vi "turn.vi"(8 "Angle":dbl=45.0 format="%#_13g", 10 "y":dbl=-1.0, 11 "RobotDriveDevRef":T1={"DevStatus"={"status"=FALSE, "code"=0, "source"=""}, "Motors[]"=[], "Square Inputs"=FALSE, "Max Output"=1.0}) -> (3 "RobotDriveDevRef dup.":T1={"DevStatus"={"status"=FALSE, "code"=0, "source"=""}, "Motors[]"=[], "Square Inputs"=FALSE, "Max Output"=1.0})   [LabVIEW 2016]
uses:
  <vilib>/Rock Robotics/WPI/RobotDrive/WPI_RobotDriveDevRef.ctl
  <vilib>/Rock Robotics/WPI/MotorControl/WPI_MotorControlDeviceRef.ctl
  <vilib>/Rock Robotics/WPI/MotorControl/WPI_MotorControlType.ctl
  <vilib>/Rock Robotics/SystemInterfaces/DIO/FPGA_DIOPWMChannel.ctl
  <vilib>/Rock Robotics/WPI/PWM/WPI_PWMDeadband.ctl
  <vilib>/Rock Robotics/WPI/RobotDrive/WPI_RobotDriveArcadeDrive_Standard(NoSaturation).vi
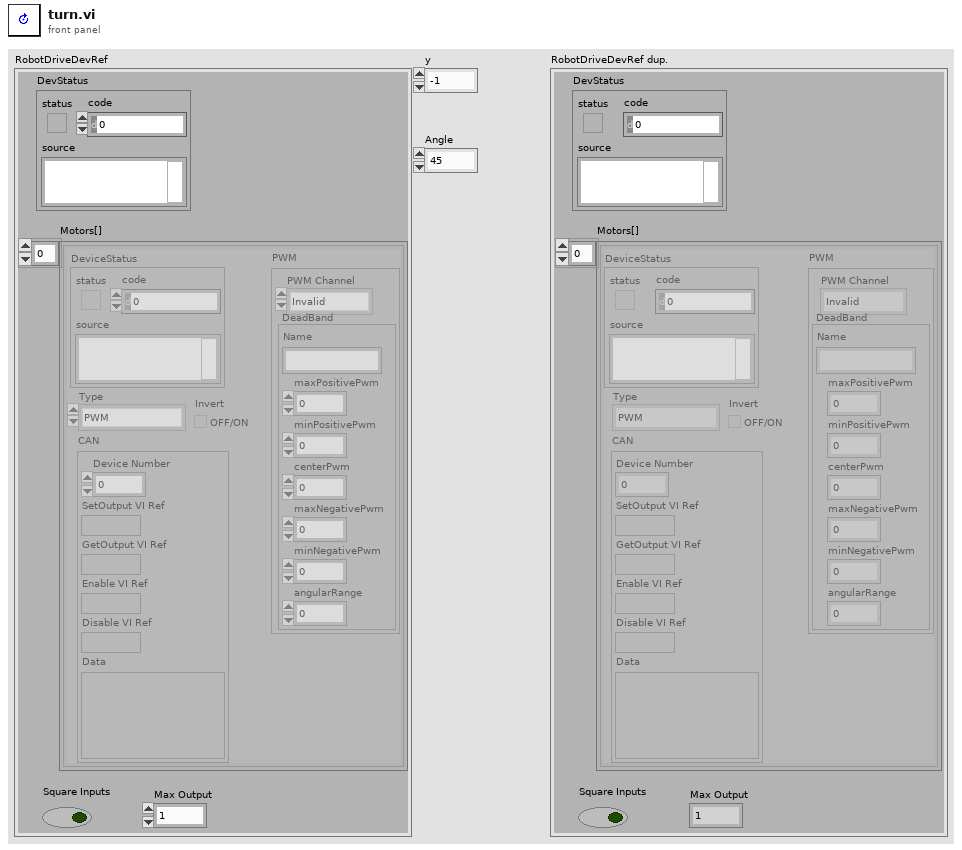
[diagram p1: front panel]
types:
  T1 = typedef "WPI_RobotDriveDevRef.ctl" = cluster{"DevStatus":errorcluster, "Motors[]":T2[], "Square Inputs":bool, "Max Output":dbl}
  T2 = typedef "WPI_MotorControlDeviceRef.ctl" = cluster{"DeviceStatus":errorcluster, "Type":T3, "PWM":cluster{"PWM Channel":T4, "DeadBand":T5}, "CAN":cluster{"Device Number":u8, "SetOutput VI Ref":variant, "GetOutput VI Ref":variant, "Enable VI Ref":variant, "Disable VI Ref":variant, "Data":variant}, "Invert":bool}
  T3 = typedef "WPI_MotorControlType.ctl" = enum16{"PWM", "CAN"}
  T4 = typedef "FPGA_DIOPWMChannel.ctl" = enum8{"PWM 0", "PWM 1", "PWM 2", "PWM 3", "PWM 4", "PWM 5", "PWM 6", "PWM 7", "PWM 8", "PWM 9", "PWM MXP 0", "PWM MXP 1", "PWM MXP 2", "PWM MXP 3", "PWM MXP 4", "PWM MXP 5", "PWM MXP 6", "PWM MXP 7", "PWM MXP 8", "PWM MXP 9", "Invalid"}
  T5 = typedef "WPI_PWMDeadband.ctl" = cluster{"Name":string, "maxPositivePwm":i32, "minPositivePwm":i32, "centerPwm":i32, "maxNegativePwm":i32, "minNegativePwm":i32, "angularRange":u16}
  T6 = typedef "WPI_GyroDevRef.ctl" = cluster{"DevStatus":errorcluster, "Analog Channel":T7, "Offset":dbl, "Gain (VoltsPerDegree/Second)":dbl, "Gyro Type":enum16{"Analog", "XRS450"}, "Handle":i32, "SPI Bus":T8, "Device Found":bool, "Sample Rate":dbl, "Calibrate On Open":bool}
  T7 = typedef "FPGA_AIChannel.ctl" = enum8{"AI 0", "AI 1", "AI 2", "AI 3", "AI MXP 0", "AI MXP 1", "AI MXP 2", "AI MXP 3", "Invalid"}
  T8 = typedef "spi_bus.ctl" = enum16{"SPI On-Board, CS0", "SPI On-Board, CS1", "SPI On-Board, CS2", "SPI On-Board, CS3", "SPI MXP", "Invalid"}
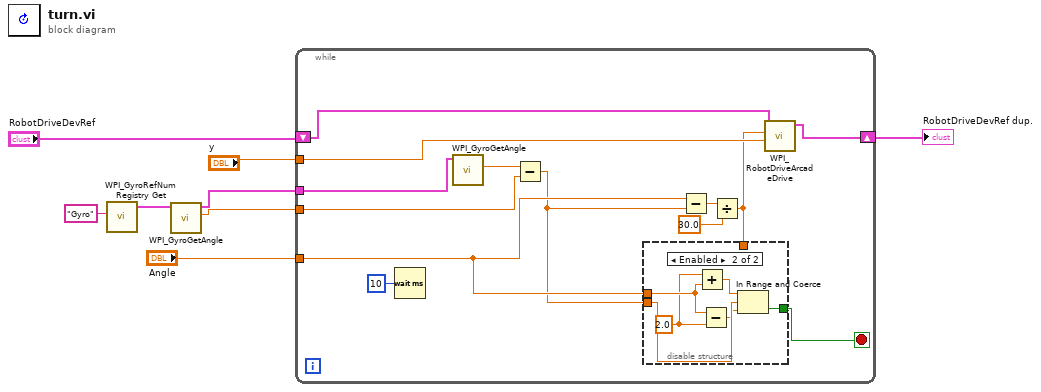
[diagram p0: block diagram]
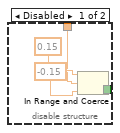
[diagram p2: hidden frame]
diagram:
  n1 = call <vilib>:"WPI_GyroRefNum Registry Get.vi"("refnum name"="Gyro") -> ("GyroDevRef"=w4:T6)  [unwired: 9 in, 1 out]
  n2 = call <vilib>:"WPI_GyroGetAngle.vi"("GyroDevRef"=w4) -> ("Angle"=w3:dbl, "GyroDevRef"=w2:T6)  [unwired: 6 in, 3 out]
  n3 = while {
    shift-right: [w20] -> w8
    shift-left: "RobotDriveDevRef" -> [w21]
    tunnel: "y" -> [w19]
    tunnel: "Angle" -> [w14]
    tunnel: w3 -> [w11]
    tunnel: w2 -> [w9]
    stop <- w18 stop-if-true
    n4 = Wait (ms)(milliseconds to wait=u32 10) -> ()  [unwired: 1 out]
    n5 = call <vilib>:"WPI_GyroGetAngle.vi"("GyroDevRef"=w9) -> ("Angle"=w10:dbl)  [unwired: 6 in, 4 out]
    n6 = Subtract(x=w10, y=w11) -> (x-y=w12:dbl)
    n7 = Subtract(x=w14, y=w12) -> (x-y=w17:dbl)
    n8 = Divide(x=w17, y=30.0) -> (x/y=w16:dbl)
    n9 = disable-structure shown="Enabled" {
      disable-tunnel: [w23 w31] -> w18
      disable-tunnel: w16 -> [w22 _]
      disable-tunnel: w12 -> [_ w30]
      disable-tunnel: w14 -> [_ w28]
      frame Disabled {
        n10 = In Range and Coerce(upper limit=0.15, x=w22, lower limit=-0.15) -> (In Range?=w23:bool)  [unwired: 1 out]
      }
      frame Enabled {
        w26 = 2.0 ("x")
        n11 = Add(x=w26, y=w28) -> (x+y=w29:dbl)
        n12 = Subtract(x=w28, y=w26) -> (x-y=w27:dbl)
        n13 = In Range and Coerce(upper limit=w29, x=w30, lower limit=w27) -> (In Range?=w31:bool)  [unwired: 1 out]
      }
    }
    n14 = call-poly <vilib>:"WPI_RobotDriveArcadeDrive.vi"("Y axis value"=w19, "X axis value"=w16, "RobotDriveDevRef"=w21) -> ("RobotDriveDevRef"=w20:T1)  [unwired: 6 in, 2 out]
  }
  "RobotDriveDevRef dup." <- w8
